vi "Config Panel.vi"(8 "error in (no error)":errorcluster, 10 "Mimic Data in":T1) -> (0 "error out":errorcluster, 1 "Mimic Picture":picture, 2 "Mimic Data out":T1)   [LabVIEW 2014, in "SeqLoop.lvlib" / "Mimico Display.lvlib"]
uses:
  Mimico Display.lvlib
  TypeDefs/Mimic Data.ctl
  TypeDefs/BG Image.ctl
  TypeDefs/mObject.ctl
  <vilib>/Utility/miscctls.llb/LVPositionTypeDef.ctl
  <vilib>/Utility/miscctls.llb/LVPointTypeDef.ctl
  <vilib>/regexp/Match Regular Expression.xnode
panel:
  in  "Open Template":bool
  in  "Save Template":bool
  in  "Select Img":string(combo)="Planilla"
  in  "BG Image":T4
  in  "Cancel":bool
  in  "Save":bool
  in  "DEL":bool
  in  "ADD":bool
  in  "Mediciones  Disponibles":i32(listbox)
  in  "mObject Data":T5 {"Ref Index." min=0 max=999; "Precision (Digits)" min=0 max=5}
  # "Medicion Seleccionada"
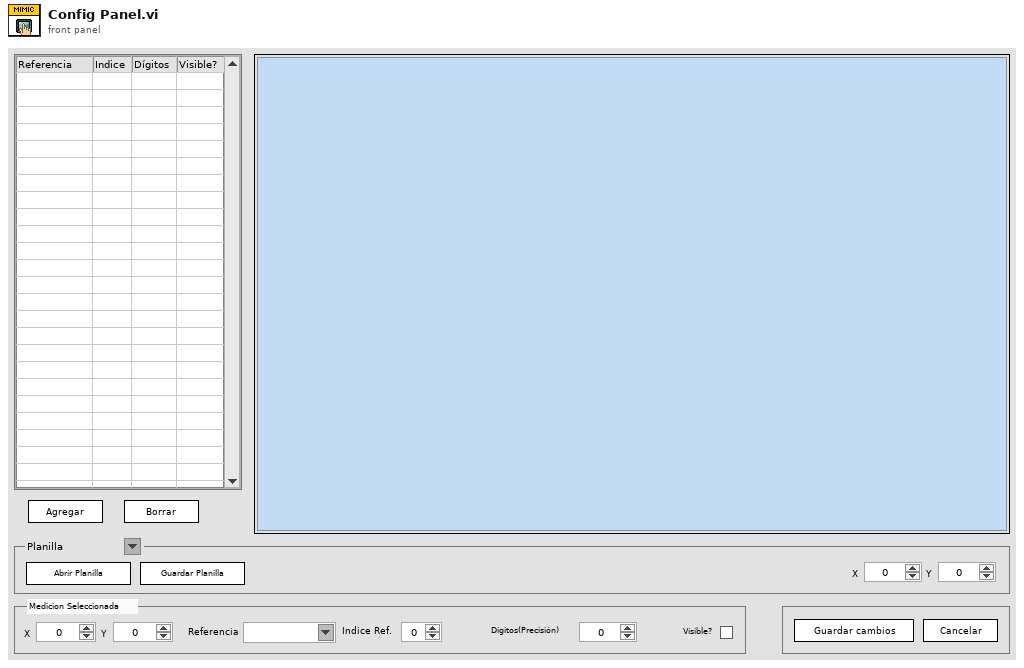
[diagram p1: front panel]
types:
  T1 = typedef "SeqLoop.lvlib/Mimico Display.lvlib/Mimic Data.ctl" = cluster{"BG Image":T2, "Mimic mObjects":T3[]}
  T2 = typedef "SeqLoop.lvlib/Mimico Display.lvlib/BG Image.ctl" = cluster{"Path":path, "point":cluster{"x":i16, "y":i16}}
  T3 = typedef "SeqLoop.lvlib/Mimico Display.lvlib/mObject.ctl" = cluster{"point":cluster{"x":i16, "y":i16}, "Precision (Digits)":i32, "Visible?":bool, "Ref":string, "Comment":string}
  T4 = cluster{"BGimage path":path, "point":cluster{"X":i16, "Y":i16}}
  T5 = cluster{"point":cluster{"X":i16, "Y":i16}, "Precision (Digits)":i32, "Visible?":bool, "Referencia":string, "Ref Index.":i32, "Comment":string, "Write":bool}
  T6 = typedef "LVPositionTypeDef.ctl" = cluster{"Left":i32, "Top":i32}
  T7 = cluster{"point":cluster{"X":i16, "Y":i16}, "Precision (Digits)":i32, "Visible?":bool, "Referencia":string, "Ref Index.":i32, "Desc.":string, "Write":bool}
  T8 = typedef "LVPointTypeDef.ctl" = cluster{"Horizontal":i16, "Vertical":i16}
  T9 = enum16{"open", "replace", "create", "open or create", "replace or create", "replace or create with confirmation"}
  T10 = typedef "eventvkey.ctl" = enum16{"ASCII", "Enter", "Return", "Shift", "Ctrl", "Alt", "Cmd", "Opt", "Caps", "NumLock", "Clear", "Break", "Up", "Down", "Left", "Right", "Insert", "Delete", "Home", "End", "PageUp", "PageDown", "Escape", "Help", "Pause", "ScrollLock", "F1", "F2", "F3", "F4", "F5", "F6", "F7", "F8", "F9", "F10", "F11", "F12", "F13", "F14", "F15", "F16", "F17", "F18", "F19", "F20", "F21", "F22", "F23", "F24", "Play", "VolumeUp", "VolumeDown", "Mute", "Two Byte Char"}
  T11 = typedef "LVMouseTypeDef.ctl" = cluster{"Mouse Position":cluster{"X":i32, "Y":i32}, "Mouse Modifiers":cluster{"Button Down":bool, "Shift Mod":bool, "Menu Mod":bool, "Option Mod":bool}}
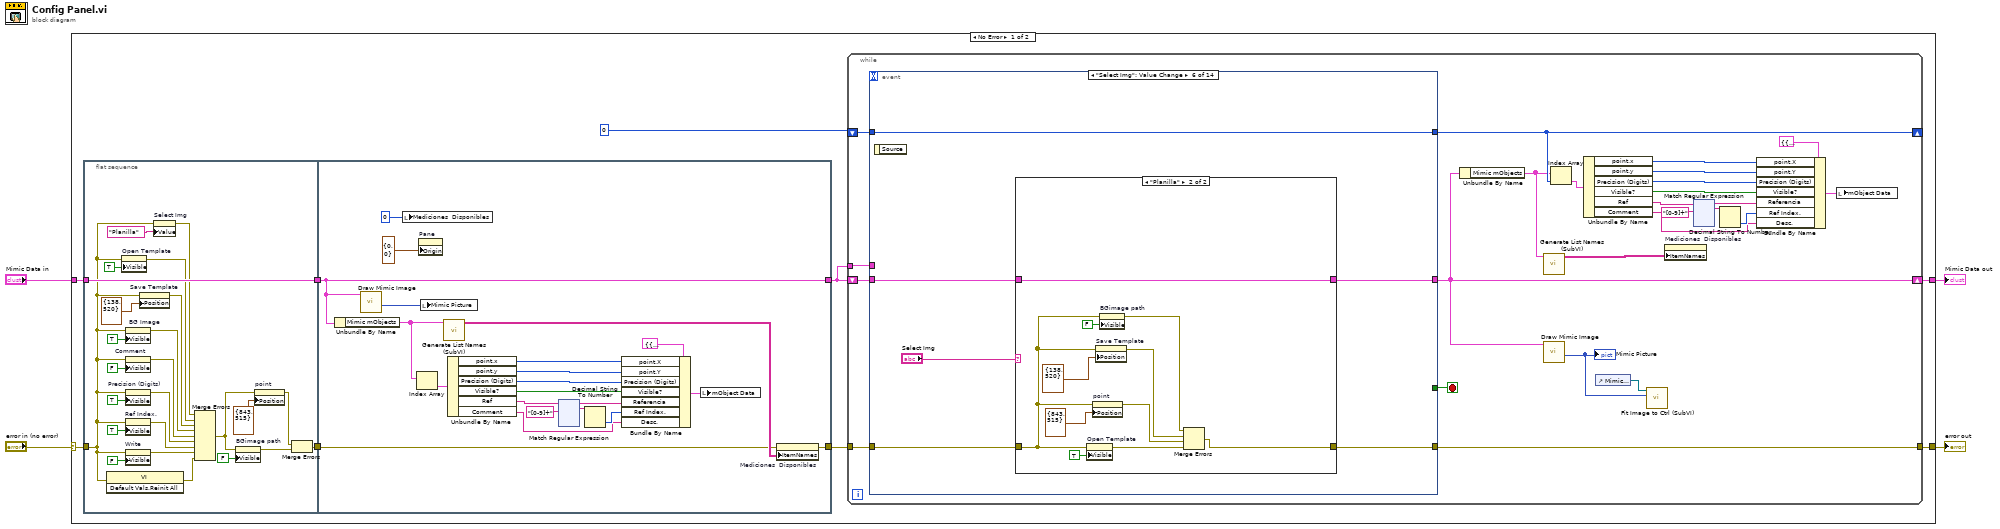
[diagram p0: block diagram]
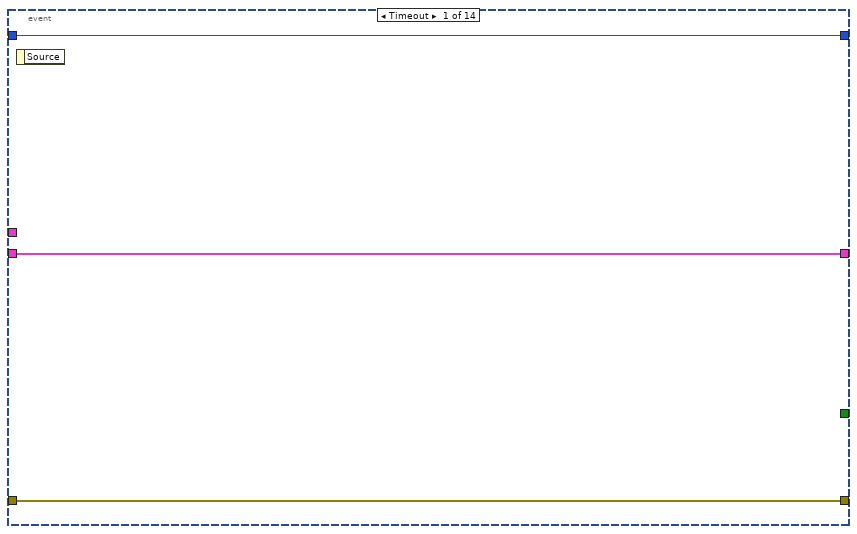
[diagram p2: hidden frame]
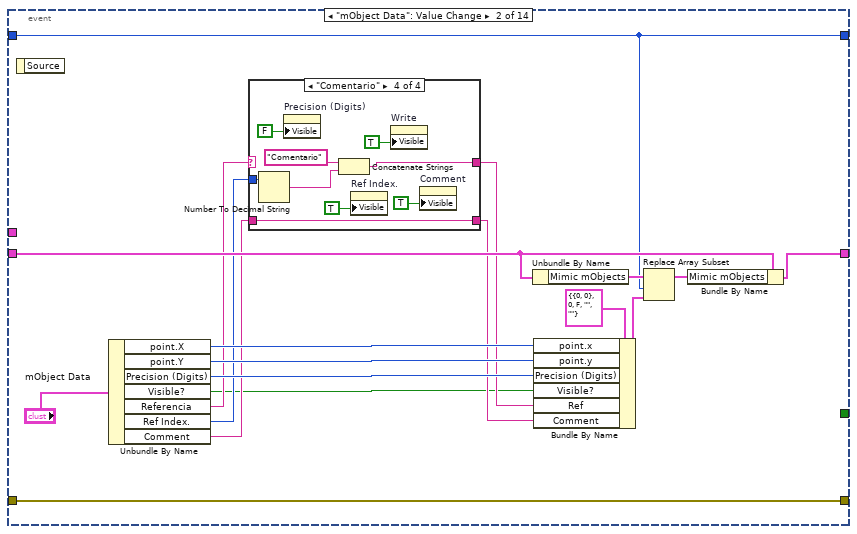
[diagram p3: hidden frame]
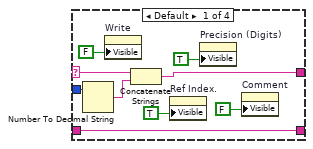
[diagram p4: hidden frame]
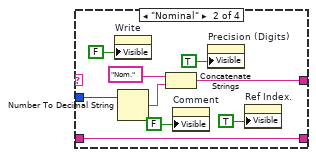
[diagram p5: hidden frame]
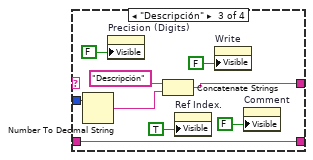
[diagram p6: hidden frame]
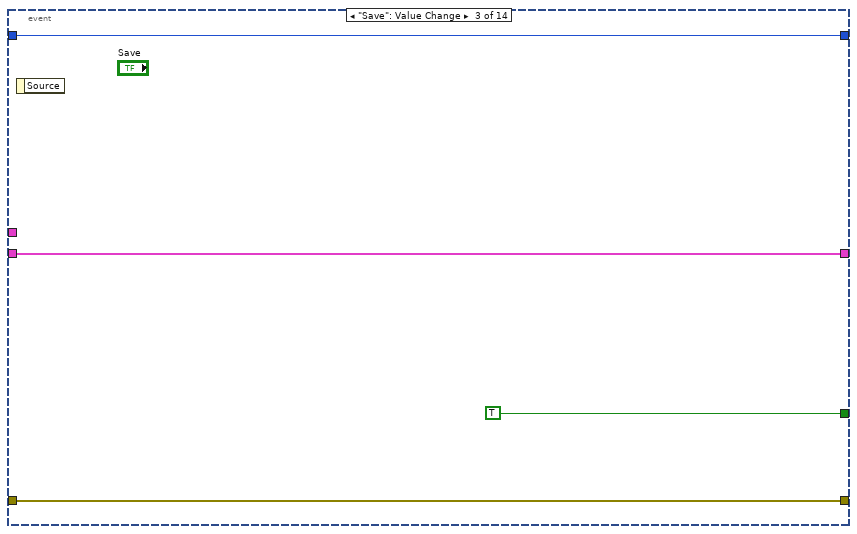
[diagram p7: hidden frame]
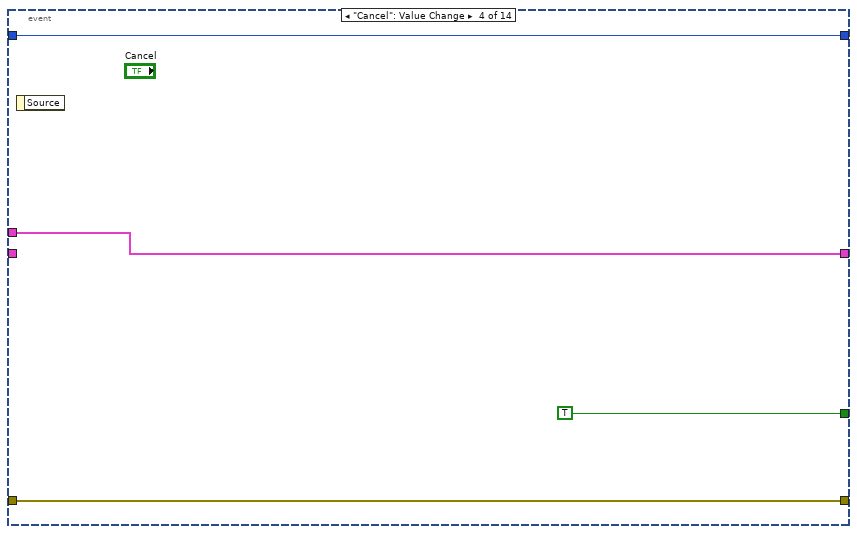
[diagram p8: hidden frame]
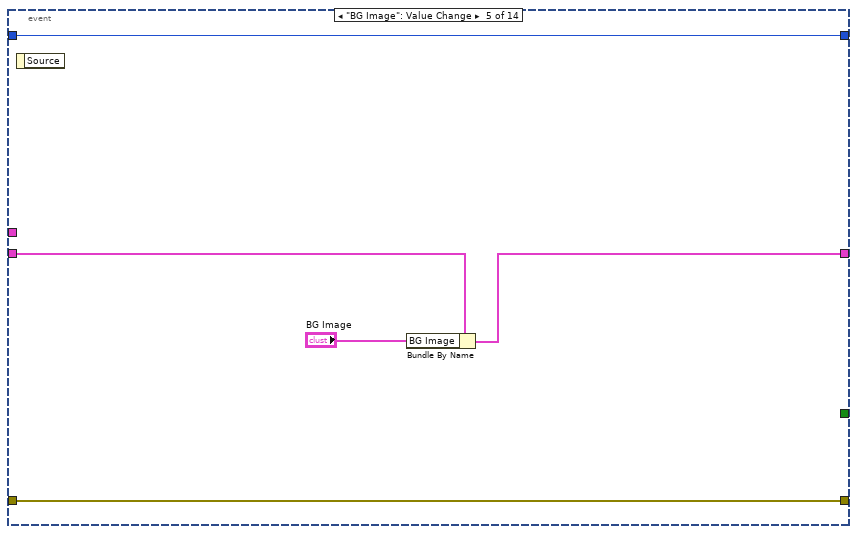
[diagram p9: hidden frame]
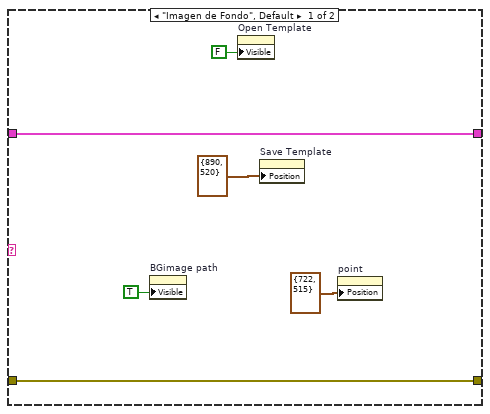
[diagram p10: hidden frame]
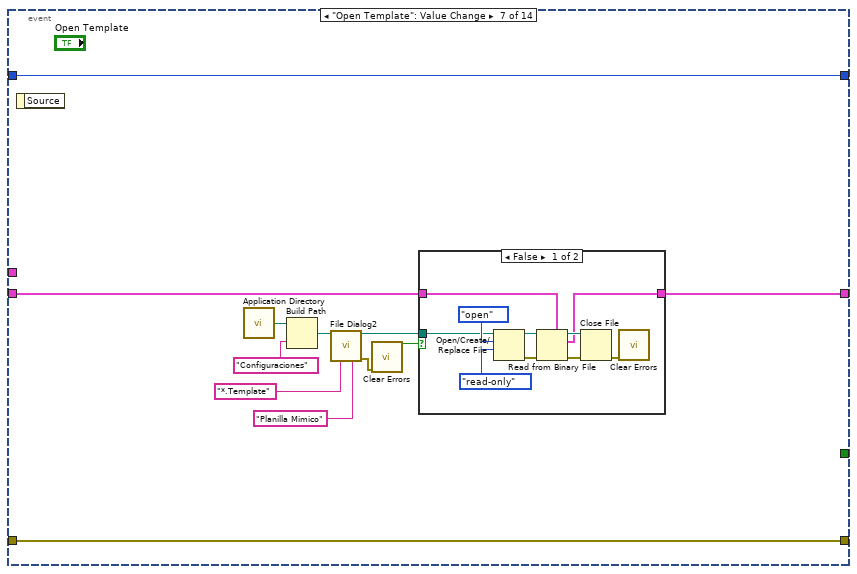
[diagram p11: hidden frame]
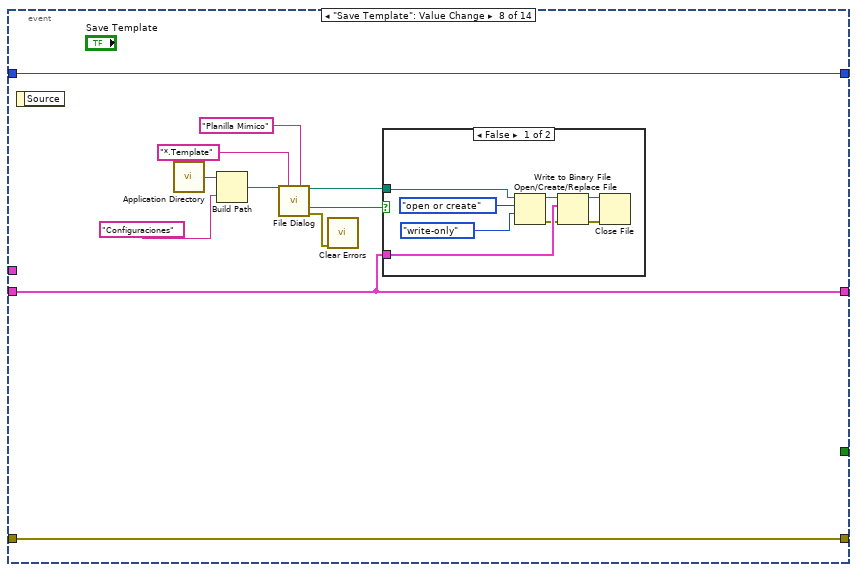
[diagram p13: hidden frame]
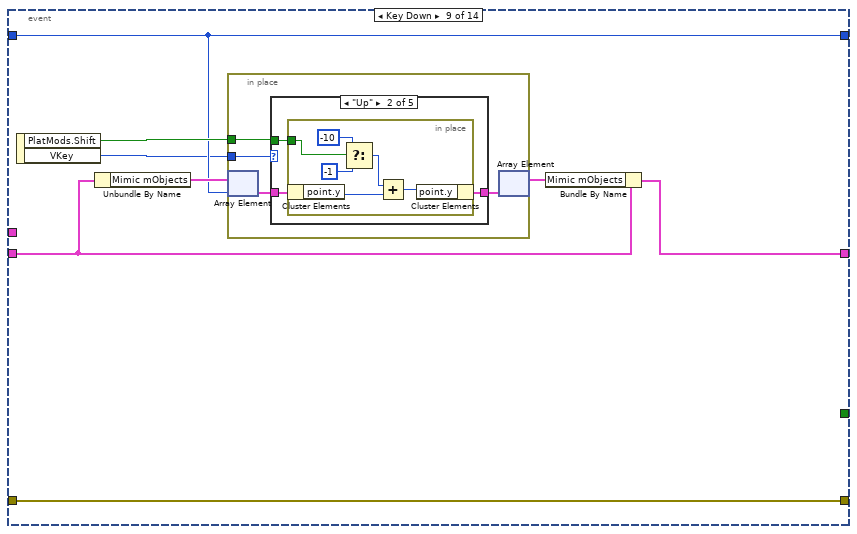
[diagram p15: hidden frame]
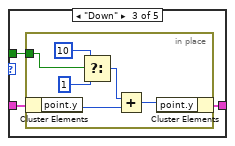
[diagram p17: hidden frame]
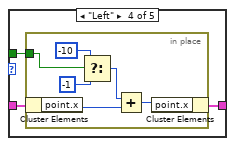
[diagram p18: hidden frame]
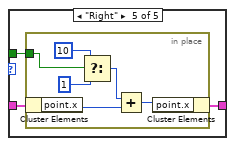
[diagram p19: hidden frame]
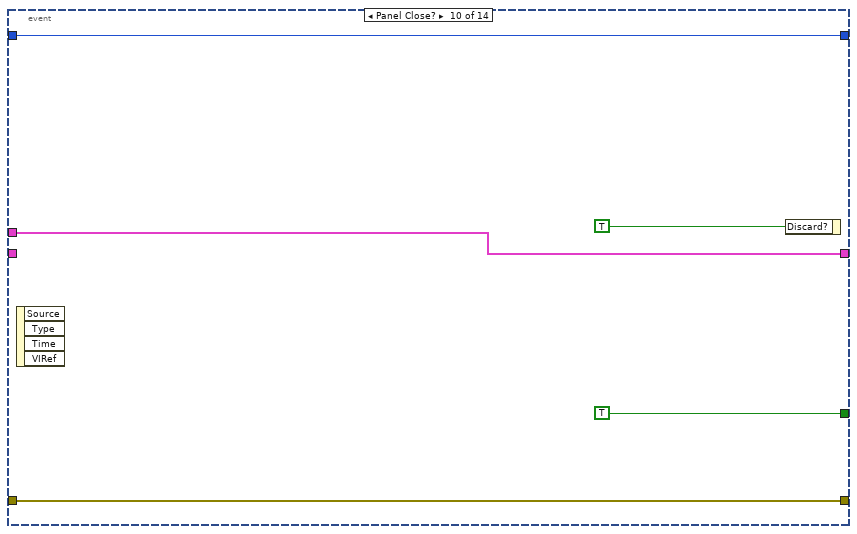
[diagram p20: hidden frame]
diagram:
  n1 = case shown="No Error" "error in (no error)" {
    selector: "error in (no error)" -> [w5 w533]
    tunnel: "Mimic Data in" -> [w9 w532]
    tunnel: [w7 w533] -> w3
    tunnel: [w6 w532] -> w2
    frame No Error {
      n2 = flat-sequence {
        tunnel: w9 -> [w38]
        tunnel: w5 -> [w20]
        tunnel: [w38] -> w13
        tunnel: [w17] -> w12
        tunnel: [w53] -> w10
        tunnel: w13 -> [w53]
        tunnel: w12 -> [w55]
        tunnel: [w54] -> w8
        frame #0 {
          n3 = invoke class="VI" method="Default Vals.Reinit All"(error in=w20) -> (error out=w29:errorcluster)  [unwired: 2 in, 2 out]
          n4 = property on="Open Template" class="Bool"(error in=w20, "Visible"=TRUE) -> (error out=w23:errorcluster)  [unwired: 1 in, 1 out]
          n5 = property on="BG Image" class="Clust (strict)"(error in=w20, "Visible"=TRUE) -> (error out=w27:errorcluster)  [unwired: 1 in, 1 out]
          n6 = property on="Comment" class="Str"(error in=w20, "Visible"=FALSE) -> (error out=w33:errorcluster)  [unwired: 1 in, 1 out]
          n7 = property on="Precision (Digits)" class="DigNum (strict)"(error in=w20, "Visible"=TRUE) -> (error out=w32:errorcluster)  [unwired: 1 in, 1 out]
          n8 = property on="Ref Index." class="DigNum (strict)"(error in=w20, "Visible"=TRUE) -> (error out=w31:errorcluster)  [unwired: 1 in, 1 out]
          n9 = property on="Write" class="Bool (strict)"(error in=w20, "Visible"=FALSE) -> (error out=w30:errorcluster)  [unwired: 1 in, 1 out]
          n10 = property on="Save Template" class="Bool"(error in=w20, "Position"=T6 {"Left"=138, "Top"=520}) -> (error out=w22:errorcluster)  [unwired: 1 in, 1 out]
          n11 = property on="Select Img" class="CmbBox"(error in=w20, "Value"="Planilla" ("Select Img")) -> (error out=w26:errorcluster)  [unwired: 1 in, 1 out]
          n12 = Merge Errors(w26, w23, w22, w27, w33, w32, w31, w30, w29) -> (w15:errorcluster)
          n13 = property on="BGimage path" class="Path"(error in=w15, "Visible"=FALSE) -> (error out=w18:errorcluster)  [unwired: 1 in, 1 out]
          n14 = property on="point" class="Clust (strict)"(error in=w15, "Position"=T6 {"Left"=843, "Top"=515}) -> (error out=w16:errorcluster)  [unwired: 1 in, 1 out]
          n15 = Merge Errors(w16, w18) -> (w17:errorcluster)
        }
        frame #1 {
          n16 = Unbundle By Name(w53) -> ("Mimic mObjects"=w57:T3[])
          n17 = call "Draw Mimic Image.vi"("Mimic Data in"=w53) -> ("Mimic Picture"=w52:picture)  [unwired: 10 in]
          n18 = local write "Mediciones  Disponibles"(0 ("Mediciones  Disponibles")) -> ()
          n19 = Index Array(array=w57) -> (element=w41:T3)  [unwired: 1 in]
          n20 = property on="Pane" class="Pane"("Origin"=T8 {"Horizontal"=0, "Vertical"=0}) -> ()  [unwired: 2 in, 2 out]
          n21 = local write "Mimic Picture"(w52) -> ()
          n22 = call "Generate List Names (SubVI).vi"("Mimic mObjects"=w57) -> ("Array"=w56:string[][])  [unwired: 10 in]
          n23 = Unbundle By Name(w41) -> ("point.x"=w50:i16, "point.y"=w49:i16, "Precision (Digits)"=w48:i32, "Visible?"=w47:bool, "Ref"=w46:string, "Comment"=w40:string)
          n24 = xnode "Match Regular Expression"("input string"=w46, "regular expression"="[0-9]+") -> ("before match"=w45:string, "whole match"=w44:string)  [unwired: 4 in, 3 out]
          n25 = Decimal String To Number(string=w44) -> (number=w43:i32)  [unwired: 2 in, 1 out]
          n26 = Bundle By Name(cluster=T7 {"point"={"X"=0, "Y"=0}, "Precision (Digits)"=0, "Visible?"=FALSE, "Referencia"="", "Ref Index."=0, "Desc."="", "Write"=FALSE} ("mObject Data 2"), "point.X"=w50, "point.Y"=w49, "Precision (Digits)"=w48, "Visible?"=w47, "Referencia"=w45, "Ref Index."=w43, "Desc."=w40) -> (w42:T7)
          n27 = local write "mObject Data"(w42) -> ()
          n28 = property on="Mediciones  Disponibles" class="MCListbox (strict)"(error in=w55, "ItemNames"=w56) -> (error out=w54:errorcluster)  [unwired: 1 in, 1 out]
        }
      }
      n29 = while {
        shift-right: [w191] -> w6
        shift-left: w10 -> [w198]
        shift-right: [w195] -> _
        shift-left: 0 ("Mediciones  Disponibles") -> [w196]
        tunnel: w10 -> [w193]
        tunnel: w8 -> [w178]
        tunnel: [w177] -> w7
        stop <- w197 stop-if-true
        n30 = event shown="[5] \"Select Img\": Value Change" {
          selector: _ -> [_ _ _ _ _ _ _ _ _ _ _ _ _ _]
          dyn-events: _ -> [_ _ _ _ _ _ _ _ _ _ _ _ _ _]
          timeout: _ -> [_ _ _ _ _ _ _ _ _ _ _ _ _ _]
          tunnel: w198 -> [w315 w333 w373 _ w379 w385 w407 w429 w455 _ w512 w517 w523 w529]
          tunnel: [w315 w330 w373 w374 w380 w387 w406 w429 w452 w497 w508 w517 w522 w528] -> w191
          tunnel: [_ _ TRUE ("stop") TRUE ("stop") _ _ _ _ _ TRUE ("stop") _ _ _ _] -> w197
          tunnel: w196 -> [w314 w329 w372 w377 w382 w388 w417 w439 w450 w501 w506 _ _ w527]
          tunnel: [w314 w329 w372 w377 w382 w388 w417 w439 w450 w501 w506 "Mediciones  Disponibles" w519 w527] -> w195
          tunnel: w193 -> [_ _ _ w374 _ _ _ _ _ w497 _ _ _ _]
          tunnel: w178 -> [w313 w319 w370 w375 w381 w384 w416 w438 w448 w498 w502 w514 w518 w526]
          tunnel: [w313 w319 w370 w375 w381 w383 w416 w438 w448 w498 w502 w514 w518 w526] -> w177
          event Timeout {
            n31 = event-data() -> ()  [unwired: 1 in, 1 out]
          }
          event "mObject Data": Value Change {
            n32 = event-data() -> ()  [unwired: 1 in, 1 out]
            n33 = Unbundle By Name("mObject Data") -> ("point.X"=w326:i16, "point.Y"=w325:i16, "Precision (Digits)"=w324:i32, "Visible?"=w316:bool, "Referencia"=w322:string, "Ref Index."=w321:i32, "Comment"=w318:string)
            n34 = case shown="\"Comentario\"" w322 {
              selector: w322 -> [w341 _ _ _]
              tunnel: w321 -> [w340 w350 w352 w361]
              tunnel: [w339 w349 w353 w362] -> w320
              tunnel: w318 -> [w335 w344 w357 w366]
              tunnel: [w335 w344 w357 w366] -> w317
              frame Default {
                n35 = Number To Decimal String(number=w340) -> (decimal integer string=w342:string)  [unwired: 1 in]
                n36 = property on="Write" class="Bool (strict)"("Visible"=FALSE) -> ()  [unwired: 2 in, 2 out]
                n37 = Concatenate Strings(w341, w342) -> (w339:string)
                n38 = property on="Ref Index." class="DigNum (strict)"("Visible"=TRUE) -> ()  [unwired: 2 in, 2 out]
                n39 = property on="Precision (Digits)" class="DigNum (strict)"("Visible"=TRUE) -> ()  [unwired: 2 in, 2 out]
                n40 = property on="Comment" class="Str"("Visible"=FALSE) -> ()  [unwired: 2 in, 2 out]
              }
              frame "Nominal" {
                n41 = property on="Write" class="Bool (strict)"("Visible"=FALSE) -> ()  [unwired: 2 in, 2 out]
                n42 = Number To Decimal String(number=w350) -> (decimal integer string=w351:string)  [unwired: 1 in]
                n43 = Concatenate Strings("Nom." ("string"), w351) -> (w349:string)
                n44 = property on="Comment" class="Str"("Visible"=FALSE) -> ()  [unwired: 2 in, 2 out]
                n45 = property on="Precision (Digits)" class="DigNum (strict)"("Visible"=TRUE) -> ()  [unwired: 2 in, 2 out]
                n46 = property on="Ref Index." class="DigNum (strict)"("Visible"=TRUE) -> ()  [unwired: 2 in, 2 out]
              }
              frame "Descripción" {
                n47 = Number To Decimal String(number=w352) -> (decimal integer string=w355:string)  [unwired: 1 in]
                n48 = property on="Precision (Digits)" class="DigNum (strict)"("Visible"=FALSE) -> ()  [unwired: 2 in, 2 out]
                n49 = Concatenate Strings("Descripción", w355) -> (w353:string)
                n50 = property on="Ref Index." class="DigNum (strict)"("Visible"=TRUE) -> ()  [unwired: 2 in, 2 out]
                n51 = property on="Write" class="Bool (strict)"("Visible"=FALSE) -> ()  [unwired: 2 in, 2 out]
                n52 = property on="Comment" class="Str"("Visible"=FALSE) -> ()  [unwired: 2 in, 2 out]
              }
              frame "Comentario" {
                n53 = Number To Decimal String(number=w361) -> (decimal integer string=w364:string)  [unwired: 1 in]
                n54 = property on="Precision (Digits)" class="DigNum (strict)"("Visible"=FALSE) -> ()  [unwired: 2 in, 2 out]
                n55 = Concatenate Strings("Comentario", w364) -> (w362:string)
                n56 = property on="Ref Index." class="DigNum (strict)"("Visible"=TRUE) -> ()  [unwired: 2 in, 2 out]
                n57 = property on="Write" class="Bool (strict)"("Visible"=TRUE) -> ()  [unwired: 2 in, 2 out]
                n58 = property on="Comment" class="Str"("Visible"=TRUE) -> ()  [unwired: 2 in, 2 out]
              }
            }
            n59 = Unbundle By Name(w333) -> ("Mimic mObjects"=w332:T3[])
            n60 = Bundle By Name(cluster=T3 {"point"={"x"=0, "y"=0}, "Precision (Digits)"=0, "Visible?"=FALSE, "Ref"="", "Comment"=""} ("mObject"), "point.x"=w326, "point.y"=w325, "Precision (Digits)"=w324, "Visible?"=w316, "Ref"=w320, "Comment"=w317) -> (w323:T3)
            n61 = Replace Array Subset(array=w332, new element=w323, index=w329) -> (w331:T3[])
            n62 = Bundle By Name(cluster=w333, "Mimic mObjects"=w331) -> (w330:T1)
          }
          event "Save": Value Change {
            n63 = event-data() -> ()  [unwired: 1 in, 1 out]
          }
          event "Cancel": Value Change {
            n64 = event-data() -> ()  [unwired: 1 in, 1 out]
          }
          event "BG Image": Value Change {
            n65 = event-data() -> ()  [unwired: 1 in, 1 out]
            n66 = Bundle By Name(cluster=w379, "BG Image"="BG Image") -> (w380:T1)
          }
          event "Select Img": Value Change {
            n67 = event-data() -> ()  [unwired: 1 in, 1 out]
            n68 = case shown="\"Planilla\"" "Select Img" {
              tunnel: w385 -> [w394 w405]
              tunnel: [w394 w405] -> w387
              tunnel: w384 -> [w391 w397]
              tunnel: [w391 w400] -> w383
              frame "Imagen de Fondo", Default {
                n69 = property on="BGimage path" class="Path"("Visible"=TRUE) -> ()  [unwired: 2 in, 2 out]
                n70 = property on="Open Template" class="Bool"("Visible"=FALSE) -> ()  [unwired: 2 in, 2 out]
                n71 = property on="Save Template" class="Bool"("Position"=T6 {"Left"=890, "Top"=520}) -> ()  [unwired: 2 in, 2 out]
                n72 = property on="point" class="Clust (strict)"("Position"=T6 {"Left"=722, "Top"=515}) -> ()  [unwired: 2 in, 2 out]
              }
              frame "Planilla" {
                n73 = property on="Open Template" class="Bool"(error in=w397, "Visible"=TRUE) -> (error out=w401:errorcluster)  [unwired: 1 in, 1 out]
                n74 = property on="point" class="Clust (strict)"(error in=w397, "Position"=T6 {"Left"=843, "Top"=515}) -> (error out=w396:errorcluster)  [unwired: 1 in, 1 out]
                n75 = property on="Save Template" class="Bool"(error in=w397, "Position"=T6 {"Left"=138, "Top"=520}) -> (error out=w402:errorcluster)  [unwired: 1 in, 1 out]
                n76 = property on="BGimage path" class="Path"(error in=w397, "Visible"=FALSE) -> (error out=w398:errorcluster)  [unwired: 1 in, 1 out]
                n77 = Merge Errors(w398, w402, w396, w401) -> (w400:errorcluster)
              }
            }
          }
          event "Open Template": Value Change {
            n78 = event-data() -> ()  [unwired: 1 in, 1 out]
            n79 = call <vilib>:"Application Directory.vi"() -> ("Application Directory"=w412:path)
            n80 = Build Path(base path=w412, name or relative path="Configuraciones") -> (appended path=w411:path)
            n81 = call "File Dialog2"("start path"=w411, "pattern (all files)"="*.Template", "pattern label"="Planilla Mimico") -> ("selected path"=w409:path, "error out"=w413:errorcluster)  [unwired: 9 in, 2 out]
            n82 = call <vilib>:"Clear Errors.vi"("error in (no error)"=w413) -> ("specific error cleared?"=w408:bool)  [unwired: 5 in, 1 out]
            n83 = case shown="False" w408 {
              tunnel: [w421 w428] -> w406
              tunnel: w407 -> [w420 w428]
              tunnel: w409 -> [w418 _]
              frame False {
                n84 = Open/Create/Replace File(file path (use dialog)=w418, operation (0:open)=T9."open", access (0:read/write)=enum16{"read/write", "read-only", "write-only"}."read-only") -> (refnum out=w426:refnum<file>, error out=w424:errorcluster)  [unwired: 3 in, 1 out]
                n85 = Read from Binary File(5:w420, 8:w424, 11:w426) -> (0:w423:errorcluster, 2:w421:T1, 3:w425:refnum<file>)  [unwired: 3 in, 1 out]
                n86 = Close File(refnum=w425, error in=w423) -> (error out=w422:errorcluster)  [unwired: 1 out]
                n87 = call <vilib>:"Clear Errors.vi"("error in (no error)"=w422) -> ()  [unwired: 5 in, 2 out]
              }
              frame True {
              }
            }
          }
          event "Save Template": Value Change {
            n88 = event-data() -> ()  [unwired: 1 in, 1 out]
            n89 = call <vilib>:"Application Directory.vi"() -> ("Application Directory"=w435:path)
            n90 = Build Path(base path=w435, name or relative path="Configuraciones") -> (appended path=w437:path)
            n91 = call "File Dialog"("start path"=w437, "pattern (all files)"="*.Template", "pattern label"="Planilla Mimico") -> ("selected path"=w430:path, "cancelled"=w433:bool, "error out"=w434:errorcluster)  [unwired: 9 in, 1 out]
            n92 = call <vilib>:"Clear Errors.vi"("error in (no error)"=w434) -> ()  [unwired: 5 in, 2 out]
            n93 = case shown="False" w433 {
              tunnel: w429 -> [w447 _]
              tunnel: w430 -> [w443 _]
              frame False {
                n94 = Open/Create/Replace File(file path (use dialog)=w443, operation (0:open)=T9."open or create", access (0:read/write)=enum16{"read/write", "read-only", "write-only"}."write-only") -> (refnum out=w444:refnum<file>, error out=w441:errorcluster)  [unwired: 3 in, 1 out]
                n95 = Write to Binary File(file (use dialog)=w444, data=w447, error in=w441) -> (refnum out=w442:refnum<file>, error out=w440:errorcluster)  [unwired: 3 in, 1 out]
                n96 = Close File(refnum=w442, error in=w440) -> ()  [unwired: 2 out]
              }
              frame True {
              }
            }
          }
          event Key Down {
            n97 = event-data() -> ("PlatMods.Shift"=w451:bool, "VKey"=w449:T10)  [unwired: 1 in]
            n98 = Unbundle By Name(w455) -> ("Mimic mObjects"=w454:T3[])
            n99 = in-place {
              in-place-border: w449 -> [w459]
              in-place-border: w451 -> [w456]
              n100 = in-place-array #1(w454, w450) -> (w458:T3)
              n101 = case shown="\"Up\"" w459 {
                tunnel: w458 -> [w460 w463 w472 w481 w490]
                tunnel: [w460 w462 w471 w480 w489] -> w457
                tunnel: w456 -> [_ w461 w470 w479 w488]
                frame Default {
                }
                frame "Up" {
                  n102 = in-place {
                    in-place-border: w461 -> [w466]
                    n103 = in-place-cluster #2(w463) -> ("point.y"=w469:i16)
                    n104 = Select(t=-10, s=w466, f=-1) -> (s? t:f=w467:i32)
                    n105 = Add(x=w467, y=w469) -> (x+y=w468:i32)
                    n106 = in-place-cluster #2("point.y"=w468) -> (w462:T3)
                  }
                }
                frame "Down" {
                  n107 = in-place {
                    in-place-border: w470 -> [w475]
                    n108 = in-place-cluster #3(w472) -> ("point.y"=w478:i16)
                    n109 = Select(t=10, s=w475, f=1) -> (s? t:f=w476:i32)
                    n110 = Add(x=w476, y=w478) -> (x+y=w477:i32)
                    n111 = in-place-cluster #3("point.y"=w477) -> (w471:T3)
                  }
                }
                frame "Left" {
                  n112 = in-place {
                    in-place-border: w479 -> [w484]
                    n113 = in-place-cluster #4(w481) -> ("point.x"=w487:i16)
                    n114 = Select(t=-10, s=w484, f=-1) -> (s? t:f=w485:i32)
                    n115 = Add(x=w485, y=w487) -> (x+y=w486:i32)
                    n116 = in-place-cluster #4("point.x"=w486) -> (w480:T3)
                  }
                }
                frame "Right" {
                  n117 = in-place {
                    in-place-border: w488 -> [w493]
                    n118 = in-place-cluster #5(w490) -> ("point.x"=w496:i16)
                    n119 = Select(t=10, s=w493, f=1) -> (s? t:f=w494:i32)
                    n120 = Add(x=w494, y=w496) -> (x+y=w495:i32)
                    n121 = in-place-cluster #5("point.x"=w495) -> (w489:T3)
                  }
                }
              }
              n122 = in-place-array #1(w457) -> (w453:T3[])  [unwired: 1 out]
            }
            n123 = Bundle By Name(cluster=w455, "Mimic mObjects"=w453) -> (w452:T1)
          }
          event Panel Close? {
            n124 = event-data() -> ()  [unwired: 1 in, 4 out]
            n125 = event-data("Discard?"=TRUE) -> ()  [unwired: 1 in, 1 out]
          }
          event "Mimic Picture": Mouse Down {
            n126 = event-data() -> ()  [unwired: 1 in, 1 out]
            n127 = property on="Mimic Picture" class="Pict"() -> ("Mouse"=w513:T11)  [unwired: 2 in, 2 out]
            n128 = Unbundle By Name(w512) -> ("Mimic mObjects"=w510:T3[])
            n129 = Unbundle By Name(w513) -> ("Mouse Position"=w505:cluster{"X":i32, "Y":i32})
            n130 = Index Array(array=w510, index=w506) -> (element=w511:T3)
            n131 = Add(x=cluster{"X":i32, "Y":i32} {"X"=-80, "Y"=-40}, y=w505) -> (x+y=w504:cluster{"X":i32, "Y":i32})
            n132 = Bundle By Name(cluster=w511, "point"=w504) -> (w507:T3)
            n133 = Replace Array Subset(array=w510, new element=w507, index=w506) -> (w509:T3[])
            n134 = Bundle By Name(cluster=w512, "Mimic mObjects"=w509) -> (w508:T1)
          }
          event "Mediciones  Disponibles": Value Change {
            n135 = event-data() -> ()  [unwired: 1 in, 1 out]
            n136 = property on="Mediciones  Disponibles" class="MCListbox (strict)"("Key Focus"=FALSE) -> ()  [unwired: 2 in, 2 out]
          }
          event "ADD": Value Change {
            n137 = event-data() -> ()  [unwired: 1 in, 1 out]
            n138 = Unbundle By Name(w523) -> ("Mimic mObjects"=w525:T3[])
            n139 = Build Array (concatenate)(w525, T3 {"point"={"x"=0, "y"=0}, "Precision (Digits)"=4, "Visible?"=TRUE, "Ref"="", "Comment"=""} ("mObject Data")) -> (w521:T3[])
            n140 = Bundle By Name(cluster=w523, "Mimic mObjects"=w521) -> (w522:T1)
            n141 = Array Size(array=w521) -> (size(s)=w520:i32)
            n142 = Decrement(x=w520) -> (x-1=w519:i32)
            n143 = local write "Mediciones  Disponibles"(w519) -> ()
          }
          event "DEL": Value Change {
            n144 = event-data() -> ()  [unwired: 1 in, 1 out]
            n145 = Unbundle By Name(w529) -> ("Mimic mObjects"=w531:T3[])
            n146 = Delete From Array(array=w531, index=w527) -> (array with subset deleted=w530:T3[])  [unwired: 1 in, 1 out]
            n147 = Bundle By Name(cluster=w529, "Mimic mObjects"=w530) -> (w528:T1)
          }
        }
        n148 = Unbundle By Name(w191) -> ("Mimic mObjects"=w192:T3[])
        n149 = call "Generate List Names (SubVI).vi"("Mimic mObjects"=w192) -> ("Array"=w194:string[][])  [unwired: 10 in]
        n150 = call "Draw Mimic Image.vi"("Mimic Data in"=w191) -> ("Mimic Picture"=w190:picture)  [unwired: 10 in]
        "Mimic Picture" <- w190
        n151 = Index Array(array=w192, index=w195) -> (element=w188:T3)
        n152 = Unbundle By Name(w188) -> ("point.x"=w186:i16, "point.y"=w185:i16, "Precision (Digits)"=w184:i32, "Visible?"=w183:bool, "Ref"=w182:string, "Comment"=w176:string)
        n153 = control-ref of="Mimic Picture"() -> (w174:refnum<vi>)
        n154 = call "Fit Image to Ctrl (SubVI).vi"("picture in"=w190, "Picture ref in"=w174) -> ()  [unwired: 10 in]
        n155 = property on="Mediciones  Disponibles" class="MCListbox (strict)"("ItemNames"=w194) -> ()  [unwired: 2 in, 2 out]
        n156 = xnode "Match Regular Expression"("input string"=w182, "regular expression"="[0-9]+") -> ("before match"=w181:string, "whole match"=w180:string)  [unwired: 4 in, 3 out]
        n157 = Decimal String To Number(string=w180) -> (number=w179:i32)  [unwired: 2 in, 1 out]
        n158 = Bundle By Name(cluster=T7 {"point"={"X"=0, "Y"=0}, "Precision (Digits)"=0, "Visible?"=FALSE, "Referencia"="", "Ref Index."=0, "Desc."="", "Write"=FALSE} ("mObject Data 2"), "point.X"=w186, "point.Y"=w185, "Precision (Digits)"=w184, "Visible?"=w183, "Referencia"=w181, "Ref Index."=w179, "Desc."=w176) -> (w187:T7)
        n159 = local write "mObject Data"(w187) -> ()
      }
    }
    frame Error {
    }
  }
  "error out" <- w3
  "Mimic Data out" <- w2
